vi "calibrated_to_raw-scalar.vi"(5 "tag_name":string, 7 "runtime":variant, 8 "error in (no error)":errorcluster, 11 "value in":dbl) -> (0 "error out":errorcluster, 3 "value out":dbl)   [LabVIEW 2015, in "lv-calibration.lvlib"]
uses:
  lv-calibration.lvlib
  _controls/error.ctl
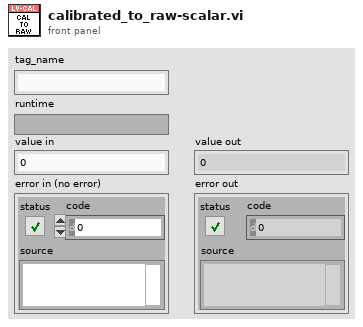
[diagram p1: front panel]
types:
  T1 = typedef "lv-calibration.lvlib/error.ctl" = enum16{"<error>", "unsupported_calibration_type", "tag_name_not_found", "duplicate_tag_names", "formula_empty"}
  T2 = typedef "lv-calibration.lvlib/runtime.ctl" = cluster{"tag_name":string, "type":T3, "offset":dbl, "slope":dbl, "formula":string, "x_points":dbl[], "y_points":dbl[]}
  T3 = typedef "lv-calibration.lvlib/type.ctl" = string
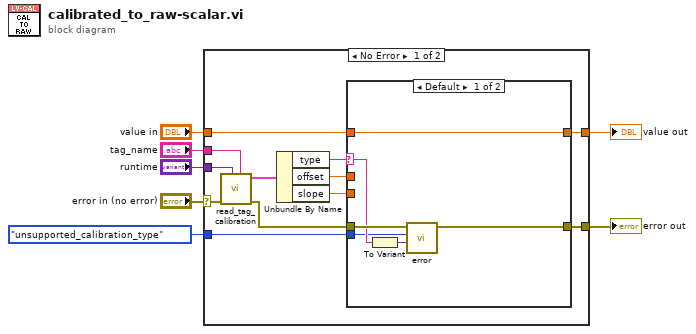
[diagram p0: block diagram]
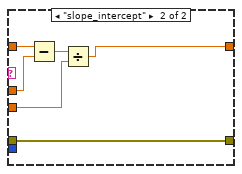
[diagram p2: hidden frame]
diagram:
  n1 = case shown="No Error" "error in (no error)" {
    selector: "error in (no error)" -> [w9 w32]
    tunnel: "value in" -> [w16 _]
    tunnel: [w15 _] -> w1
    tunnel: [w14 w32] -> w2
    tunnel: error."unsupported_calibration_type" ("error") -> [w13 _]
    tunnel: "runtime" -> [w11 _]
    tunnel: "tag_name" -> [w10 _]
    frame No Error {
      n2 = call "read_tag_calibration.vi"("tag_name"=w10, "runtime"=w11, "error in (no error)"=w9) -> ("error out"=w8:errorcluster, "calibration"=w12:T2)  [unwired: 7 in]
      n3 = Unbundle By Name(w12) -> ("type"=w19:T3, "offset"=w18:dbl, "slope"=w17:dbl)
      n4 = case shown="Default" w19 {
        selector: w19 -> [w23 _]
        tunnel: w8 -> [w24 w31]
        tunnel: w18 -> [_ w27]
        tunnel: w17 -> [_ w26]
        tunnel: w16 -> [w25 w30]
        tunnel: [w25 w28] -> w15
        tunnel: [w20 w31] -> w14
        tunnel: w13 -> [w21 _]
        frame Default {
          n5 = To Variant(anything=w23) -> (Variant=w22:variant)
          n6 = call "error.vi"("data"=w22, "error"=w21, "error in (no error)"=w24) -> ("error out"=w20:errorcluster)  [unwired: 8 in]
        }
        frame "slope_intercept" {
          n7 = Subtract(x=w30, y=w27) -> (x-y=w29:dbl)
          n8 = Divide(x=w29, y=w26) -> (x/y=w28:dbl)
        }
      }
    }
    frame Error {
    }
  }
  "error out" <- w2
  "value out" <- w1
